vi "InitDevice.vi"(0 "设备类型":u32(ring)=3 items=["PCI5121"=1, "PCI9810"=2, "USBCAN1"=3, "USBCAN2"=4, "PCI9820"=5, "PCI5110"=7, "PC104CAN"=11, "CANETUDP"=12, "PCI9840B"=14, "PC104C2"=15, "PCI9820I"=16, "CANETTCP"=17, "PCIE9221"=24, "PCI5010U"=19, "USBCAN_E_U"=20, "USBCAN_2E_U"=21, "PCI5020U"=22], 1 "ID(Hex 高位有效)":string="40A", 2 "DeviceInd":u32, 3 "CANInd":u32, 4 "Baud":u32(ring)=11 caption="波特率" items=["5Kbps", "10Kbps", "20Kbps", "40Kbps", "50Kbps", "80Kbps", "100Kbps", "125Kbps", "200Kbps", "250Kbps", "400Kbps", "500Kbps", "666Kbps", "800Kbps", "1000Kbps"], 5 "错误输入（无错误）":errorcluster, 7 "滤波":bool) -> (14 "DeviceType":u32, 15 "Result":bool, 16 "DeviceIndex":u32, 17 "CANIndex":u32, 19 "错误输出":errorcluster)   [LabVIEW 2013]
uses:
  ControlCAN.dll
panel:
  out "输出簇":T1 {"验收码" format="%x"; "屏蔽码" format="%08x"}
  in  "VCI_INIT_CONFIG":T1={"验收码"=0, "屏蔽码"=4294967295, "Reserved"=0, "滤波方式"=1, "Timing0"=0, "Timing1"=20, "模式"=0} {"模式" items=["正常", "只听"]; "滤波方式" items=["双滤波", "单滤波"]; "屏蔽码" format="0x%08x"; "验收码" format="0x%08x"; "Timing1" format="%x"; "Timing0" format="%x"; "Reserved" format="%x"}
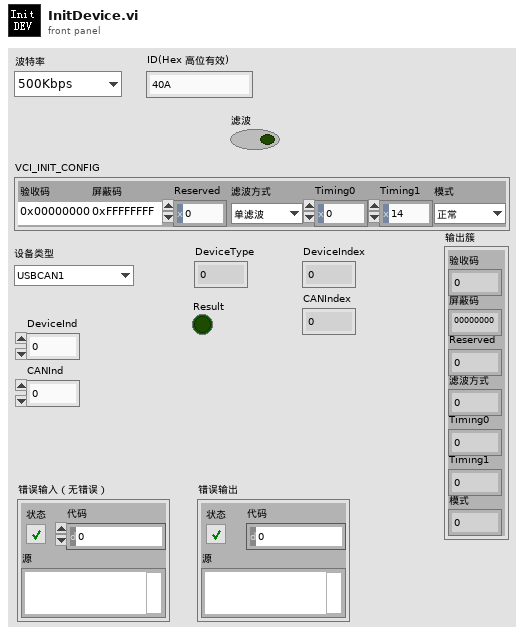
[diagram p1: front panel]
types:
  T1 = cluster{"验收码":u32, "屏蔽码":u32, "Reserved":u32, "滤波方式":u8, "Timing0":u8, "Timing1":u8, "模式":u8}
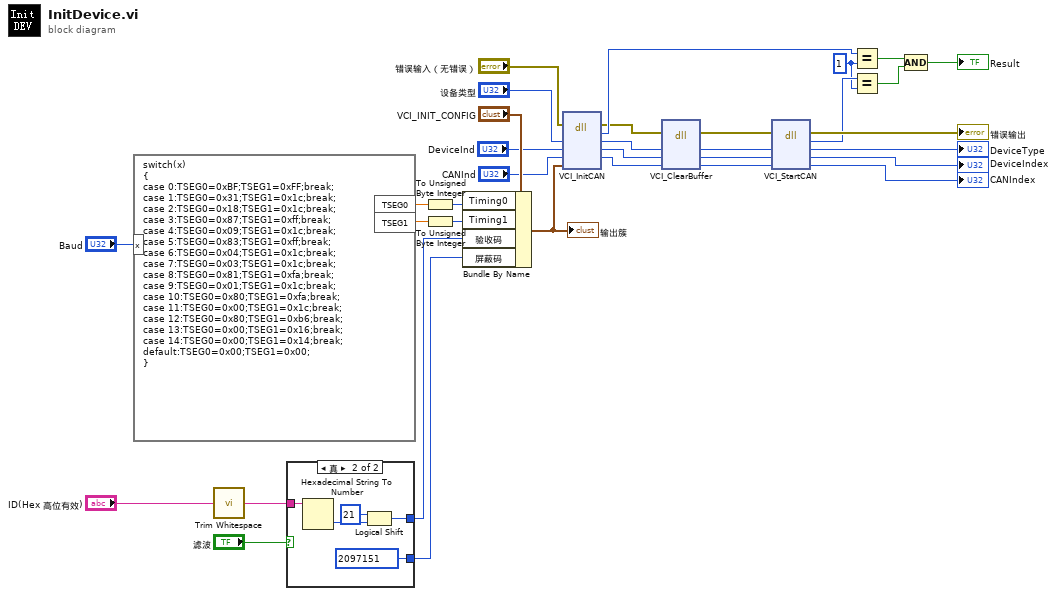
[diagram p0: block diagram]
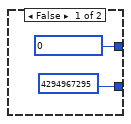
[diagram p2: hidden frame]
diagram:
  w19 = u32 1 ("y")
  n1 = formula code="switch(x)\n{ \ncase 0:TSEG0=0xBF;TSEG1=0xFF;break;\ncase 1:TSEG0=0x31;TSEG1=0x1c;break;\ncase 2:TSEG0=0x18;TSEG1=0x1c;break;\ncase 3:TSEG0=0x87;TSEG1=0xff;break;\ncase 4:TSEG0=0x09;TSEG1=0x1c;break;\ncase 5:TSEG0=0x83;TSEG1=0xff;break;\ncase 6:TSEG0=0x04;TSEG1=0x1c;break;\ncase 7:TSEG0=0x03;TSEG1=0x1c;break;\ncase 8:TSEG0=0x81;TSEG1=0xfa;break;\ncase 9:TSEG0=0x01;TSEG1=0x1c;break;\ncase 10:TSEG0=0x80;TSEG1=0xfa;break;\ncase 11:TSEG0=0x00;TSEG1=0x1c;break;\ncase 12:TSEG0=0x80;TSEG1=0xb6;break;\ncase 13:TSEG0=0x00;TSEG1=0x16;break;\ncase 14:TSEG0=0x00;TSEG1=0x14;break;\ndefault:TSEG0=0x00;TSEG1=0x00;\n}"("x"="Baud") -> ("TSEG0"=w30:dbl, "TSEG1"=w29:dbl)
  n2 = call <vilib>:"Trim Whitespace.vi"("string"="ID(Hex 高位有效)") -> ("trimmed string"=w17:string)  [unwired: 1 in]
  n3 = case shown="真" "滤波" {
    tunnel: w17 -> [_ w39]
    tunnel: [u32 0 ("验收码") w38] -> w9
    tunnel: [u32 4294967295 ("屏蔽码") u32 2097151 ("屏蔽码")] -> w16
    frame False {
    }
    frame True {
      n4 = Hexadecimal String To Number(string=w39) -> (number=w41:u32)  [unwired: 2 in, 1 out]
      n5 = Logical Shift(y=i8 21, x=w41) -> (x << y=w38:u32)
    }
  }
  n6 = To Unsigned Byte Integer(number=w30) -> (unsigned 8bit integer=w27:u8)
  n7 = To Unsigned Byte Integer(number=w29) -> (unsigned 8bit integer=w28:u8)
  n8 = Bundle By Name(cluster="VCI_INIT_CONFIG", "Timing0"=w27, "Timing1"=w28, "验收码"=w9, "屏蔽码"=w16) -> (w26:T1)
  "输出簇" <- w26
  n9 = dll-call lib="PTH1`abs E桌面休眠电流方案休眠电流源码20181130\nInstrumentCANControlCAN.dll" fn="VCI_InitCAN"(error in="错误输入（无错误）", "DeviceType"="设备类型", "DeviceInd"="DeviceInd", "CANInd"="CANInd", "VCI_INIT_CONFIG"=w26) -> (error out=w11:errorcluster, w14:u32, "DeviceType"=w13:u32, "DeviceInd"=w6:u32, "CANInd"=w5:u32)  [unwired: 3 in, 1 out]
  n10 = dll-call lib="PTH1`abs E桌面休眠电流方案休眠电流源码20181130\nInstrumentCANControlCAN.dll" fn="VCI_ClearBuffer"(error in=w11, "DeviceType"=w13, "DeviceInd"=w6, "CANInd"=w5) -> (error out=w10:errorcluster, "DeviceType"=w12:u32, "DeviceInd"=w4:u32, "CANInd"=w3:u32)  [unwired: 2 in, 2 out]
  n11 = dll-call lib="PTH1`abs E桌面休眠电流方案休眠电流源码20181130\nInstrumentCANControlCAN.dll" fn="VCI_StartCAN"(error in=w10, "DeviceType"=w12, "DeviceInd"=w4, "CANInd"=w3) -> (error out=→"错误输出":errorcluster, w21:u32, "DeviceType"=→"DeviceType":u32, "DeviceInd"=→"DeviceIndex":u32, "CANInd"=→"CANIndex":u32)  [unwired: 2 in, 1 out]
  n12 = Equal?(x=w14, y=w19) -> (x = y?=w25:bool)
  n13 = Equal?(x=w21, y=w19) -> (x = y?=w20:bool)
  n14 = Compound Arithmetic op=AND(w25, w20) -> (→"Result":bool)
